vi "Receive Message.vi"(0 "ICanCommunicate In":refnum<class "ICanCommunicate.lvclass">, 1 "Timeout in ms (-1)":i32, 5 "ToProcessQueue":T2, 11 "Error In":errorcluster) -> (4 "ICanCommunicate Out":refnum<class "ICanCommunicate.lvclass">, 6 "Message":T1, 10 "Timed Out?":bool, 15 "Error Out":errorcluster)   [LabVIEW 2023, in "ICanCommunicate.lvclass"]
doc: "Allows process to check its queue for pending messages."
uses:
  ICanCommunicate.lvclass
  ToProcessQueue.ctl
  Message.ctl
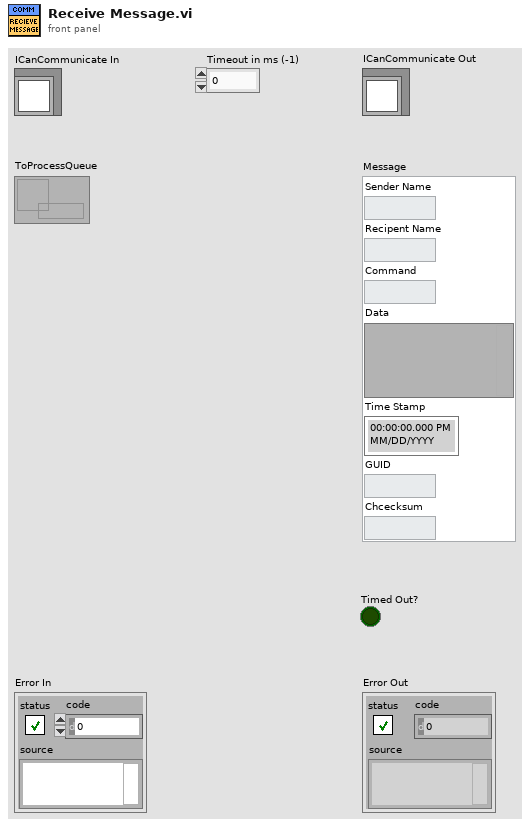
[diagram p1: front panel]
types:
  T1 = typedef "ICanCommunicate.lvclass/Message.ctl" = cluster{"Sender Name":string, "Recipent Name":string, "Command":string, "Data":variant, "Time Stamp":timestamp, "GUID":string, "Chcecksum":string}
  T2 = typedef "ICanCommunicate.lvclass/ToProcessQueue.ctl" = refnum<queue>
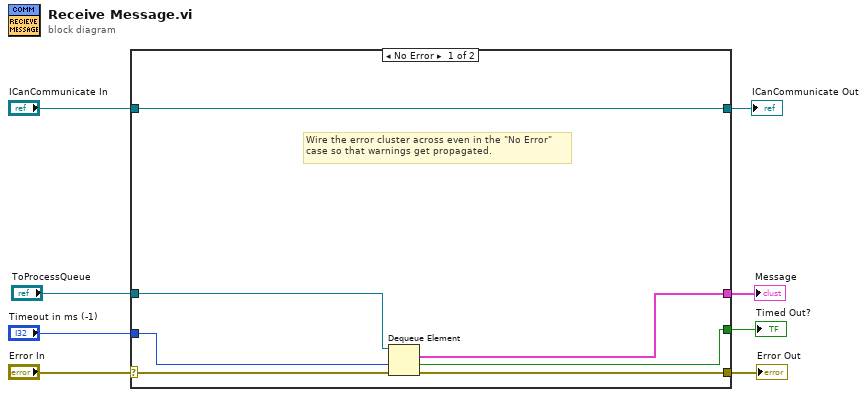
[diagram p0: block diagram]
diagram:
  n1 = case shown="No Error" "Error In" {
    selector: "Error In" -> [w14 w17]
    tunnel: [w13 w17] -> w7
    tunnel: [w15 w16] -> w5
    tunnel: "ICanCommunicate In" -> [w15 w16]
    tunnel: "Timeout in ms (-1)" -> [w12 _]
    tunnel: "ToProcessQueue" -> [w11 _]
    tunnel: [w10 _] -> w2
    tunnel: [w9 _] -> w1
    frame No Error {
      # "Wire the error cluster across even in the \"No Error\"\ncase so that warnings get propagated."
      n2 = Dequeue Element(queue=w11, timeout in ms (-1)=w12, error in (no error)=w14) -> (element=w10:T1, timed out?=w9:bool, error out=w13:errorcluster)  [unwired: 1 out]
    }
    frame Error {
    }
  }
  "Error Out" <- w7
  "ICanCommunicate Out" <- w5
  "Message" <- w2
  "Timed Out?" <- w1
